vi "runCommunications.vi"(8 "error in (no error)":errorcluster, 11 "Boot in":refnum<class "Boot.lvclass">) -> (0 "error out":errorcluster, 3 "Boot out":refnum<class "Boot.lvclass">)   [LabVIEW 2016, in "Boot.lvclass"]
uses:
  Boot.lvclass
  Boot.lvclass/Boot.ctl
  Communicator/M1M3SAL/M1M3SAL.lvclass
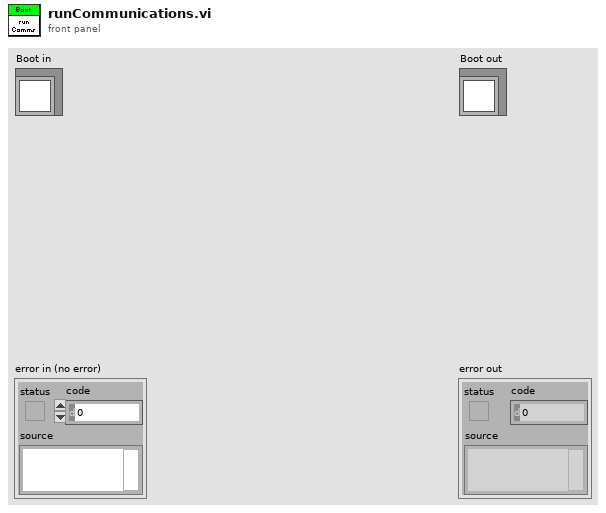
[diagram p1: front panel]
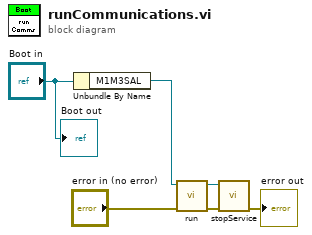
[diagram p0: block diagram]
diagram:
  n1 = Unbundle By Name("Boot in") -> ("M1M3SAL"=w1:refnum<class "M1M3SAL.lvclass">)
  n2 = call "run.vi"("error in (no error)"="error in (no error)", "M1M3SAL in"=w1) -> ("error out"=w5:errorcluster, "M1M3SAL out"=w6:refnum<class "M1M3SAL.lvclass">)  [unwired: 8 in]
  n3 = call "stopService.vi"("error in (no error)"=w5, "M1M3SAL in"=w6) -> ("error out"=→"error out":errorcluster)  [unwired: 8 in, 1 out]
  "Boot out" <- "Boot in"
